vi "ao_waveform_lite.vi"() -> ()   [LabVIEW 2020]
uses:
  <vilib>/measure/NI_MABase.lvlib
panel:
  in  "Offset":dbl
  in  "signal type":T1(ring) caption="Signal Type"
  out "error out":errorcluster caption="错误输出"
  in  "Frequency":dbl=1000.0 format="%#.6g"
  in  "Amplitude":dbl=5.0 format="%.3f"
  out "波形图":waveform(dbl)(graph)
  in  "AoCycle":u32
  in  "SamplePeriod(ns)":u32=10000
  in  "Chan":u8
  in  "DevIndex":i32
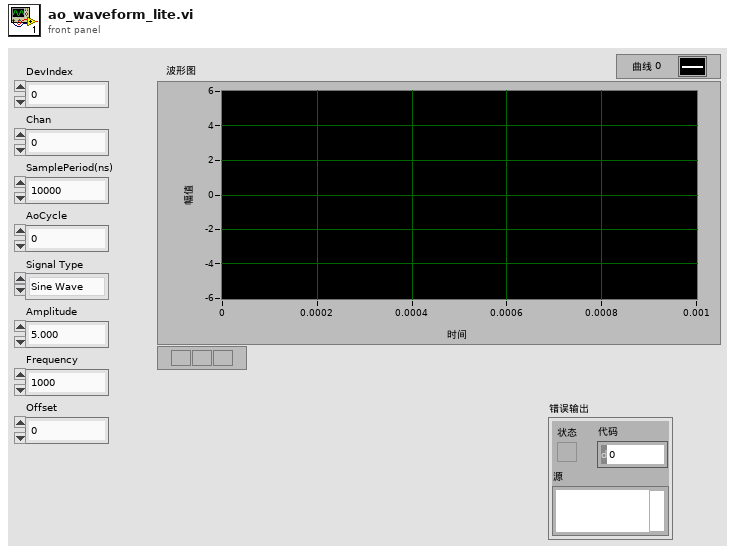
[diagram p1: front panel]
types:
  T1 = enum16{"Sine Wave", "Triangle Wave", "Square Wave", "Sawtooth Wave"}
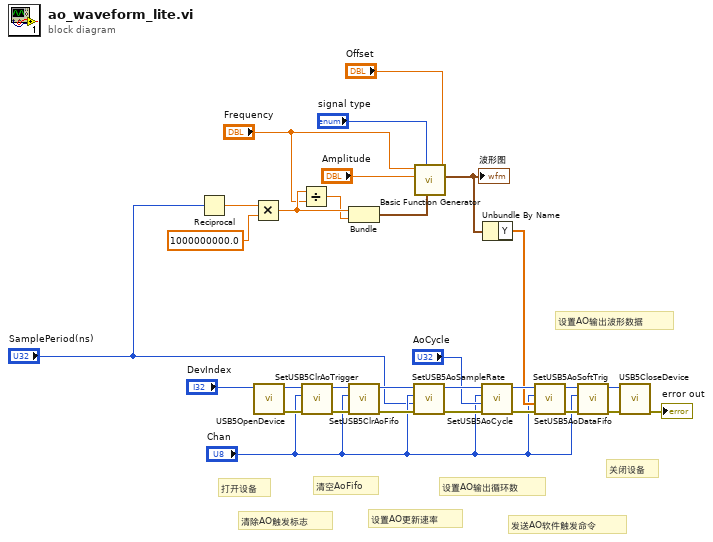
[diagram p0: block diagram]
diagram:
  # "设置AO输出波形数据"
  # "关闭设备"
  # "发送AO软件触发命令"
  # "设置AO输出循环数"
  # "设置AO更新速率"
  # "清空AoFifo"
  # "清除AO触发标志"
  # "打开设备"
  n1 = Reciprocal(x="SamplePeriod(ns)") -> (1/x=w30:dbl)
  n2 = Multiply(x=w30, y=1000000000.0) -> (x*y=w27:dbl)
  n3 = call "USB5OpenDevice.vi"("DevIndex"="DevIndex") -> ("error out"=w6:errorcluster, "DevIndex Out"=w3:i32)  [unwired: 9 in]
  n4 = Divide(x=w27, y="Frequency") -> (x/y=w26:dbl)
  n5 = call "SetUSB5ClrAoTrigger.vi"("错误输入（无错误）"=w6, "Chan"="Chan", "DevIndex"=w3) -> ("错误输出"=w5:errorcluster, "DevIndex Out"=w4:i32)  [unwired: 7 in]
  n6 = Bundle(w27, w26) -> (w29:cluster{dbl, dbl})  [unwired: 1 in]
  n7 = call "SetUSB5ClrAoFifo.vi"("错误输入（无错误）"=w5, "Chan"="Chan", "DevIndex"=w4) -> ("错误输出"=w9:errorcluster, "DevIndex Out"=w10:i32)  [unwired: 7 in]
  n8 = call "SetUSB5AoSampleRate.vi"("错误输入（无错误）"=w9, "SamplePeriod(ns)"="SamplePeriod(ns)", "Chan"="Chan", "DevIndex"=w10) -> ("错误输出"=w21:errorcluster, "DevIndex Out"=w22:i32)  [unwired: 6 in]
  n9 = call <vilib>:"Basic Function Generator.vi"("offset"="Offset", "sampling info"=w29, "signal type"="signal type", "amplitude"="Amplitude", "frequency"="Frequency") -> ("signal out"=w12:waveform(dbl))  [unwired: 4 in, 2 out]
  "波形图" <- w12
  n10 = call "SetUSB5AoCycle.vi"("错误输入（无错误）"=w21, "AoCycle"="AoCycle", "Chan"="Chan", "DevIndex"=w22) -> ("错误输出"=w19:errorcluster, "DevIndex Out"=w18:i32)  [unwired: 6 in]
  n11 = Unbundle By Name(w12) -> ("Y"=w11:dbl[])
  n12 = call "SetUSB5AoDataFifo.vi"("错误输入（无错误）"=w19, "Voltage"=w11, "Chan"="Chan", "DevIndex"=w18) -> ("错误输出"=w16:errorcluster, "DevIndex Out"=w17:i32)  [unwired: 6 in]
  n13 = call "SetUSB5AoSoftTrig.vi"("错误输入（无错误）"=w16, "Chan"="Chan", "DevIndex"=w17) -> ("错误输出"=w14:errorcluster, "DevIndex Out"=w15:i32)  [unwired: 7 in]
  n14 = call "USB5CloseDevice.vi"("错误输入（无错误）"=w14, "DevIndex"=w15) -> ("error out"=→"error out":errorcluster)  [unwired: 8 in, 1 out]
